vi "Unit Test - Add VI Reference Case.vi"() -> ()   [LabVIEW 2020]
uses:
  _csmHelper/API/Create From VI Reference.vi
  _csmHelper/Properties/Read States.vi
  _csmHelper/API/Open Front Panel.vi
  _csmHelper/API/Start Undo.vi
  _csmHelper/API/Add VI Reference Case.vi
  _csmHelper/API/Stop Undo.vi
  _csmHelper/API/Save Instrument.vi
  _csmHelper/API/Destroy.vi
  _csmHelper/CSM-Helper.lvclass
panel:
  out "error out":errorcluster
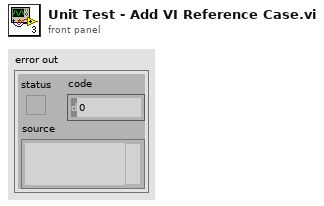
[diagram p1: front panel]
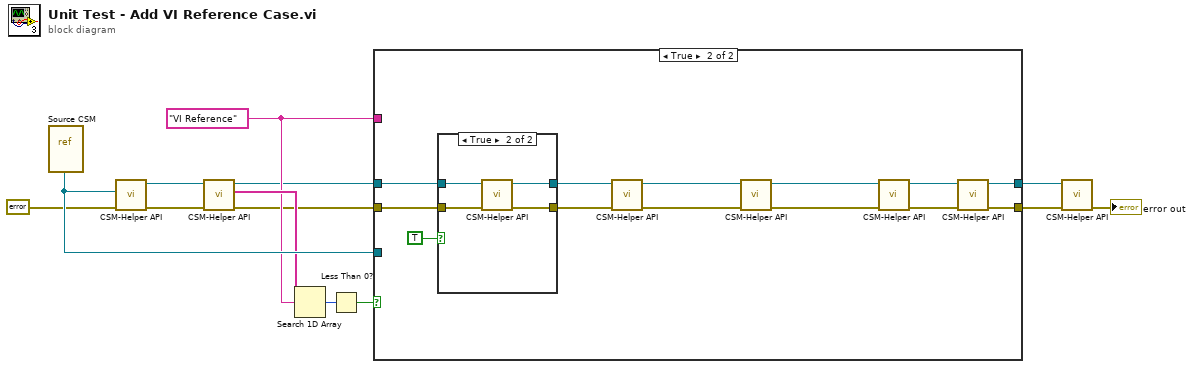
[diagram p0: block diagram]
diagram:
  w8 = "VI Reference" ("element")
  n1 = vi-ref "Source CSM.vi"() -> (w13:refnum<vi>)
  n2 = call-poly "CSM-Helper API.vi"("error in (no error)"=errorcluster {"status"=FALSE, "code"=0, "source"=""}, "VI"=w13) -> ("error out"=w2:errorcluster, "CSM-Helper.lvclass"=w3:refnum<class "CSM-Helper.lvclass">)  [unwired: 8 in]
  n3 = call-poly "CSM-Helper API.vi"("error in (no error)"=w2, "CSM-Helper in"=w3) -> ("error out"=w6:errorcluster, "Value"=w10:string[], "CSM-Helper out"=w5:refnum<class "CSM-Helper.lvclass">)  [unwired: 7 in]
  n4 = Search 1D Array(1D array=w10, element=w8) -> (index of element=w4:i32)  [unwired: 1 in]
  n5 = Less Than 0?(x=w4) -> (x < 0?=w7:bool)
  n6 = case shown="True" w7 {
    tunnel: w5 -> [w14 w28]
    tunnel: w6 -> [w15 w19]
    tunnel: w8 -> [_ _]
    tunnel: [w15 w22] -> w11
    tunnel: [w14 w24] -> w9
    tunnel: w13 -> [_ _]
    frame False {
    }
    frame True {
      n7 = case shown="True" TRUE ("Show FP?") {
        tunnel: w28 -> [w29 w34]
        tunnel: [w29 w33] -> w21
        tunnel: [w30 w32] -> w20
        tunnel: w19 -> [w30 w31]
        frame False {
        }
        frame True {
          n8 = call-poly "CSM-Helper API.vi"("error in (no error)"=w31, "CSM-Helper in"=w34) -> ("error out"=w32:errorcluster, "CSM-Helper out"=w33:refnum<class "CSM-Helper.lvclass">)  [unwired: 8 in]
        }
      }
      n9 = call-poly "CSM-Helper API.vi"("error in (no error)"=w20, "CSM-Helper in"=w21) -> ("error out"=w26:errorcluster, "CSM-Helper out"=w27:refnum<class "CSM-Helper.lvclass">)  [unwired: 8 in]
      n10 = call-poly "CSM-Helper API.vi"("error in (no error)"=w26, "CSM-Helper in"=w27) -> ("error out"=w17:errorcluster, "CSM-Helper out"=w18:refnum<class "CSM-Helper.lvclass">)  [unwired: 8 in]
      n11 = call-poly "CSM-Helper API.vi"("error in (no error)"=w17, "CSM-Helper in"=w18) -> ("error out"=w23:errorcluster, "CSM-Helper out"=w25:refnum<class "CSM-Helper.lvclass">)  [unwired: 8 in]
      n12 = call-poly "CSM-Helper API.vi"("error in (no error)"=w23, "CSM-Helper in"=w25) -> ("error out"=w22:errorcluster, "CSM-Helper out"=w24:refnum<class "CSM-Helper.lvclass">)  [unwired: 8 in]
    }
  }
  n13 = call-poly "CSM-Helper API.vi"("error in (no error)"=w11, "CSM-Helper in"=w9) -> ("error out"=→"error out":errorcluster)  [unwired: 8 in, 1 out]
